vi "Demo.vi"() -> ()   [LabVIEW 2012, in "Gradient PieChart.lvclass"]
uses:
  Gradient PieChart.lvclass
  Info.ctl
panel:
  in  "radius":i16=100
  in  "pixel center":cluster{"horizontal":i16, "vertical":i16}={"horizontal"=220, "vertical"=120} caption="Circle Center"
  out "Grad PieChart":picture
  in  "InfoArray":T1[](array[typedef])=[{"Value"=12.0, "Name"="Item One", "NameTxtColor"=16860, "Color Segement"=[16448250, 16860]}, {"Value"=32.0, "Name"="Item Two", "NameTxtColor"=16723200, "Color Segement"=[16448250, 16723200]}, {"Value"=50.0, "Name"="Item Three", "NameTxtColor"=0, "Color Segement"=[16448250, 0]}]
  in  "origin":cluster{"x":i16, "y":i16}={"x"=5, "y"=5} caption="原点"
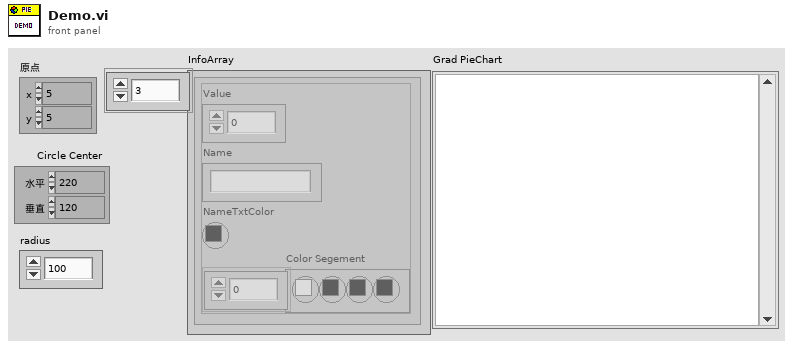
[diagram p1: front panel]
types:
  T1 = typedef "Gradient PieChart.lvclass/Info.ctl" = cluster{"Value":dbl, "Name":string, "NameTxtColor":u32, "Color Segement":u32[]}
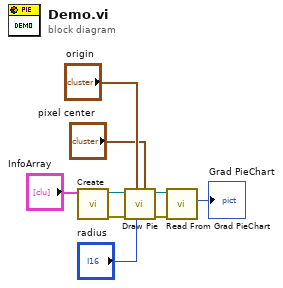
[diagram p0: block diagram]
diagram:
  n1 = call "Create.vi"("InfoArray"="InfoArray") -> ("error out"=w6:errorcluster, "Gradient PieChart 输出"=w7:refnum<class "Gradient PieChart.lvclass">)  [unwired: 9 in]
  n2 = call "Draw Pie.vi"("pixel center"="pixel center", "radius"="radius", "Legends Orin"="origin", "error in (no error)"=w6, "Gradient PieChart 输入"=w7) -> ("error out"=w2:errorcluster, "Gradient PieChart 输出"=w3:refnum<class "Gradient PieChart.lvclass">)  [unwired: 5 in]
  n3 = call "Read From Grad PieChart.vi"("error in (no error)"=w2, "Gradient PieChart输入"=w3) -> ("Grad PieChart"=→"Grad PieChart":picture)  [unwired: 7 in, 2 out]
